vi "ZMQ_mmWave_Create.vi"(8 "error in (no error)":errorcluster, 10 "endpoint":string, 11 "reference in":refnum<class "ZMQ_mmWave.lvclass">) -> (0 "error out":errorcluster, 3 "reference out":refnum<class "ZMQ_mmWave.lvclass">)   [LabVIEW 2019, in "CommandResponse communication.lvlib" / "ZMQ_mmWave.lvclass"]
doc: "Constructor."
uses:
  ZMQ_mmWave.lvclass
  C:/Program Files/National Instruments/LabVIEW 2019/vi.lib/addons/_AddQ/G#Object/G#Object.lvclass
  C:/Barkhausen mmWave radar/Development/LV/Barkhausen mmWave hardware control/Host/Intertarget communication/ZMQ_slave_class/ZMQ_slave.lvclass
  <vilib>/addons/_AddQ/G#Object/G#Object.lvclass
  Host/Intertarget communication/ZMQ_slave_class/ZMQ_slave.lvclass
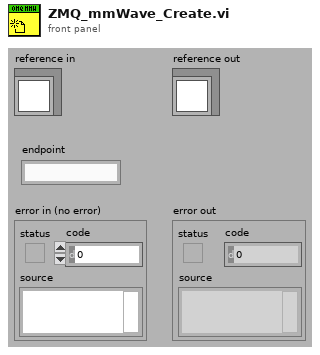
[diagram p1: front panel]
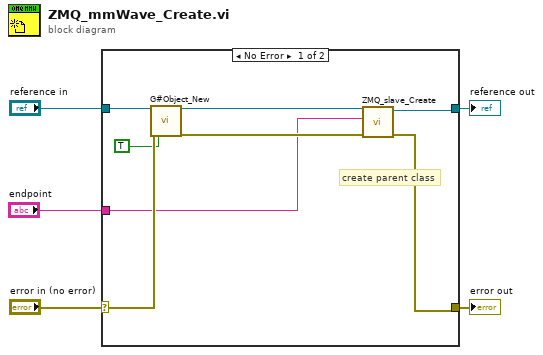
[diagram p0: block diagram]
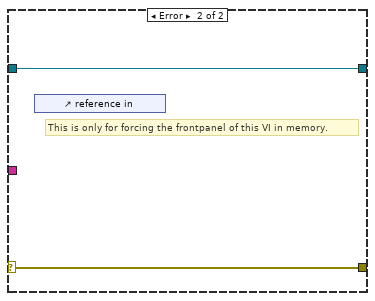
[diagram p2: hidden frame]
diagram:
  n1 = case shown="No Error" "error in (no error)" {
    selector: "error in (no error)" -> [w12 w15]
    tunnel: [w7 w15] -> w4
    tunnel: [w8 w14] -> w2
    tunnel: "reference in" -> [w13 w14]
    tunnel: "endpoint" -> [w6 _]
    frame No Error {
      # "create parent class"
      n2 = call <vilib>:"G#Object_New.vi"("reference in"=w13, "error in (no error)"=w12, "user counter (T)?"=TRUE ("User Counter")) -> ("reference out"=w10:refnum<class "ZMQ_mmWave.lvclass">, "error out"=w9:errorcluster)  [unwired: 14 in, 1 out]
      n3 = call "ZMQ_slave_Create.vi"("error in (no error)"=w9, "endpoint"=w6, "reference in"=w10) -> ("error out"=w7:errorcluster, "reference out"=w8:refnum<class "ZMQ_mmWave.lvclass">)  [unwired: 7 in]
    }
    frame Error {
      # "This is only for forcing the frontpanel of this VI in memory."
      n4 = control-ref of="reference in"() -> ()  [unwired: 1 out]
    }
  }
  "error out" <- w4
  "reference out" <- w2
